vi "ShiftToggle.vi"(9 "Right":bool, 11 "Left":bool) -> (3 "Zone Shift":bool)   [LabVIEW 2013]
uses:
  Common Code/Change Detect Boolean.vi
panel:
  out "Right State":dbl
  out "Left State":dbl
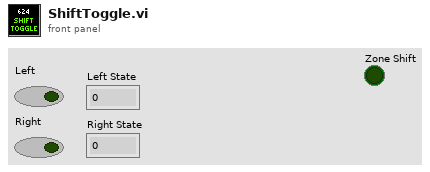
[diagram p1: front panel]
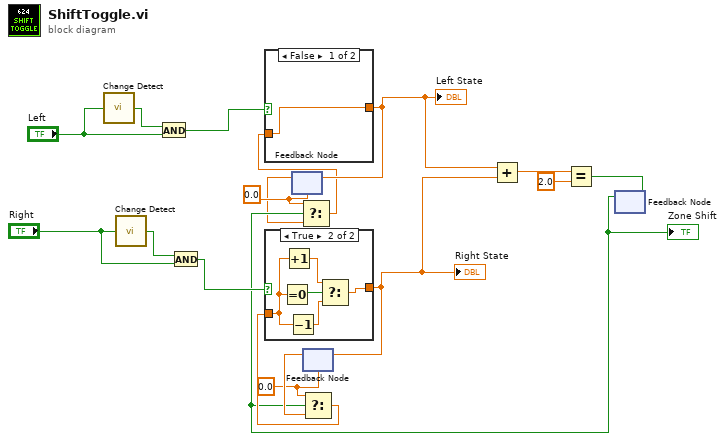
[diagram p0: block diagram]
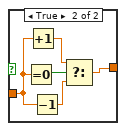
[diagram p3: hidden frame]
diagram:
  w5 = 0.0 ("t")
  w4 = 0.0
  n1 = call-poly "Change Detect.vi"("In"="Left") -> ("Changed?"=w18:bool)
  n2 = call-poly "Change Detect.vi"("In"="Right") -> ("Changed?"=w15:bool)
  n3 = And(x=w18, y="Left") -> (x .and. y?=w16:bool)
  n4 = And(x=w15, y="Right") -> (x .and. y?=w13:bool)
  n5 = feedback #1(w4) -> (w2:dbl)
  n6 = feedback #2(w5) -> (w8:dbl)
  n7 = feedback #3() -> (w3:bool)  [unwired: 1 in]
  "Zone Shift" <- w3
  n8 = Select(t=w4, s=w3, f=w2) -> (s? t:f=w1:dbl)
  n9 = case shown="False" w16 {
    tunnel: w1 -> [w19 w22]
    tunnel: [w19 w20] -> w12
    frame False {
    }
    frame True {
      n10 = Equal To 0?(x=w22) -> (x = 0?=w24:bool)
      n11 = Increment(x=w22) -> (x+1=w23:dbl)
      n12 = Decrement(x=w22) -> (x-1=w21:dbl)
      n13 = Select(t=w23, s=w24, f=w21) -> (s? t:f=w20:dbl)
    }
  }
  "Left State" <- w12
  n14 = feedback-in #1(w12) -> ()
  n15 = Select(t=w5, s=w3, f=w8) -> (s? t:f=w7:dbl)
  n16 = case shown="True" w13 {
    tunnel: w7 -> [w25 w28]
    tunnel: [w25 w26] -> w9
    frame False {
    }
    frame True {
      n17 = Equal To 0?(x=w28) -> (x = 0?=w30:bool)
      n18 = Increment(x=w28) -> (x+1=w29:dbl)
      n19 = Decrement(x=w28) -> (x-1=w27:dbl)
      n20 = Select(t=w29, s=w30, f=w27) -> (s? t:f=w26:dbl)
    }
  }
  "Right State" <- w9
  n21 = feedback-in #2(w9) -> ()
  n22 = Add(x=w12, y=w9) -> (x+y=w11:dbl)
  n23 = Equal?(x=w11, y=2.0) -> (x = y?=w6:bool)
  n24 = feedback-in #3(w6) -> ()
